vi "Unsubscribe.vi"(0 "STOMP in":refnum<class "STOMP.lvclass">, 2 "Subscription Id":u64, 5 "error in (no error)":errorcluster, 6 "Receipt?":bool) -> (14 "STOMP out":refnum<class "STOMP.lvclass">, 19 "error out":errorcluster)   [LabVIEW 2017, in "LabVIEW STOMP.lvlib" / "STOMP.lvclass"]
uses:
  STOMP.lvclass
  Typedefs/Type_ClientFrame.ctl
  Typedefs/Type_ClientFrameType.ctl
  Typedefs/Type_FrameHeader.ctl
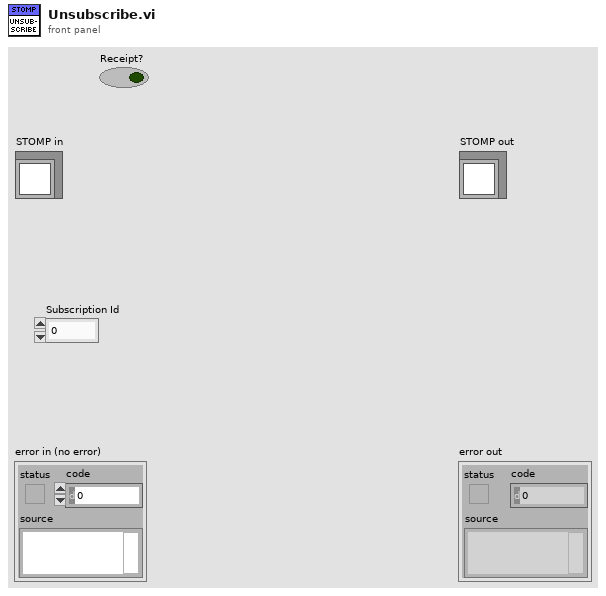
[diagram p1: front panel]
types:
  T1 = typedef "LabVIEW STOMP.lvlib/STOMP.lvclass/Type_FrameHeader.ctl" = cluster{"Header":string, "Value":string}
  T2 = typedef "LabVIEW STOMP.lvlib/STOMP.lvclass/Type_ClientFrameType.ctl" = enum16{"Undefined", "SEND", "SUBSCRIBE", "UNSUBSCRIBE", "BEGIN", "COMMIT", "ABORT", "ACK", "NACK", "DISCONNECT"}
  T3 = typedef "LabVIEW STOMP.lvlib/STOMP.lvclass/Type_ClientFrame.ctl" = cluster{"Type":T2, "Headers":T1[], "Body":string}
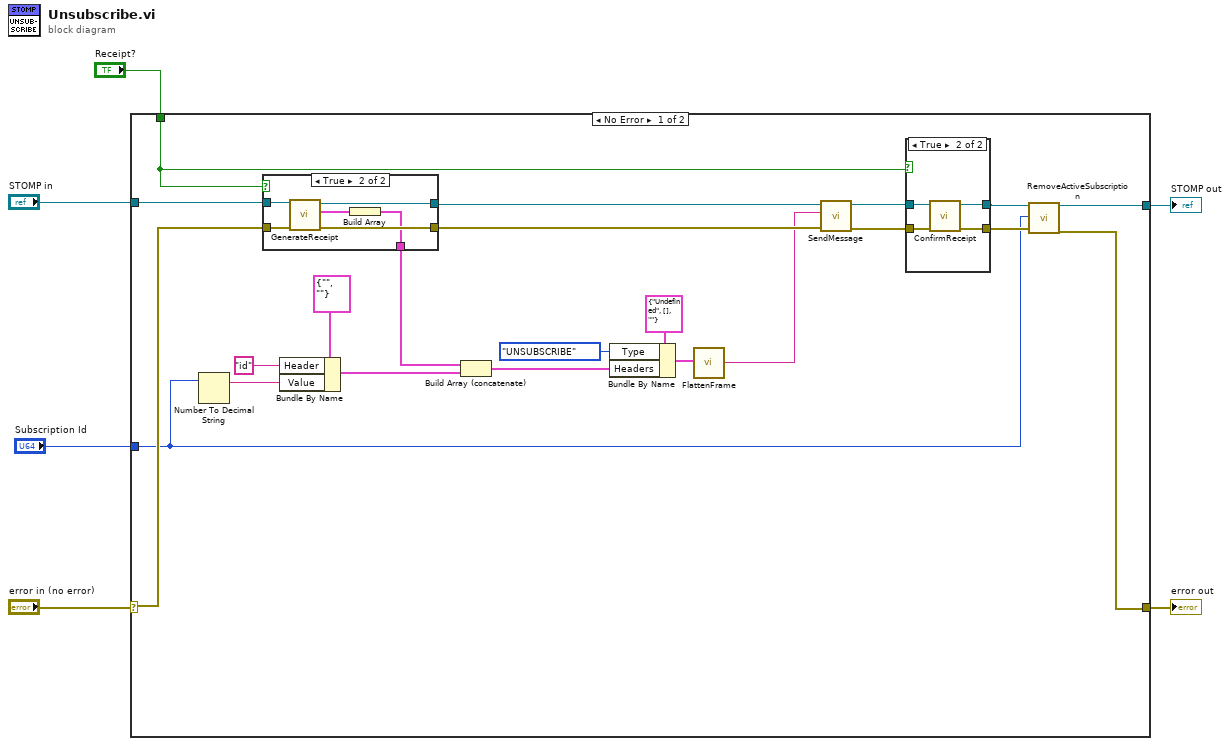
[diagram p0: block diagram]
diagram:
  n1 = case shown="No Error" "error in (no error)" {
    selector: "error in (no error)" -> [w8 w44]
    tunnel: [w22 w44] -> w5
    tunnel: [w21 w43] -> w3
    tunnel: "STOMP in" -> [w18 w43]
    tunnel: "Receipt?" -> [w19 _]
    tunnel: "Subscription Id" -> [w7 _]
    frame No Error {
      n2 = Number To Decimal String(number=w7) -> (decimal integer string=w11:string)  [unwired: 1 in]
      n3 = case shown="True" w19 {
        tunnel: [w30 w36] -> w25
        tunnel: [w29 w35] -> w26
        tunnel: [_ w33] -> w14
        tunnel: w18 -> [w30 w32]
        tunnel: w8 -> [w29 w31]
        frame False {
        }
        frame True {
          n4 = call-dynamic "GenerateReceipt.vi"("error in (no error)"=w31, "STOMP in"=w32) -> ("error out"=w35:errorcluster, "Receipt Header"=w34:T1, "STOMP out"=w36:refnum<class "STOMP.lvclass">)  [unwired: 7 in]
          n5 = Build Array(w34) -> (w33:T1[])
        }
      }
      n6 = Bundle By Name(cluster=T1 {"Header"="", "Value"=""}, "Header"="id", "Value"=w11) -> (w10:T1)
      n7 = Build Array (concatenate)(w14, w10) -> (w9:T1[])
      n8 = Bundle By Name(cluster=T3 {"Type"=enum."Undefined", "Headers"=[], "Body"=""} ("Client Frame"), "Type"=Type_ClientFrameType."UNSUBSCRIBE", "Headers"=w9) -> (w16:T3)
      n9 = call "FlattenFrame.vi"("Client Frame"=w16) -> ("flattened frame"=w20:string)  [unwired: 18 in]
      n10 = call-dynamic "SendMessage.vi"("error in (no error)"=w26, "data in"=w20, "STOMP in"=w25) -> ("error out"=w27:errorcluster, "STOMP out"=w28:refnum<class "STOMP.lvclass">)  [unwired: 7 in]
      n11 = case shown="True" w19 {
        tunnel: w28 -> [w37 w42]
        tunnel: w27 -> [w38 w41]
        tunnel: [w38 w40] -> w23
        tunnel: [w37 w39] -> w24
        frame False {
        }
        frame True {
          n12 = call-dynamic "ConfirmReceipt.vi"("error in (no error)"=w41, "STOMP in"=w42) -> ("error out"=w40:errorcluster, "STOMP out"=w39:refnum<class "STOMP.lvclass">)  [unwired: 8 in]
        }
      }
      n13 = call-dynamic "RemoveActiveSubscription.vi"("STOMP in"=w24, "id"=w7, "error in (no error)"=w23) -> ("STOMP out"=w21:refnum<class "STOMP.lvclass">, "error out"=w22:errorcluster)  [unwired: 15 in]
    }
    frame Error {
    }
  }
  "error out" <- w5
  "STOMP out" <- w3
